vi "7903 Reference Clock Config.vi"(8 "error in":errorcluster, 9 "reference clock index":u8, 10 "ref clk frequency":u64, 11 "fpga interface in":refnum<k20>) -> (0 "error out":errorcluster, 3 "fpga interface out":refnum<k20>)   [LabVIEW 2023, in "PXIe-7903 Aurora Example Host.lvlib"]
uses:
  PXIe-7903 Aurora Example Host.lvlib
  <resource>/objmgr/niflexrioapiClock.rc
  Program Files/NI/LVAddons/flexrioiia/1/instr.lib/FlexRIO/API/Host/v1/NI FlexRIO API v1.lvlib
  <vilib>/ErrorRing/Error Ring.xnode
  <vilib>/Utility/error.llb/Error Cluster From Error Code.vi
  Program Files/NI/LVAddons/flexrioiia/1/instr.lib/FlexRIO/API/Host/v1/NI FlexRIO/API/Get Property Reference - Fpga Small.vi
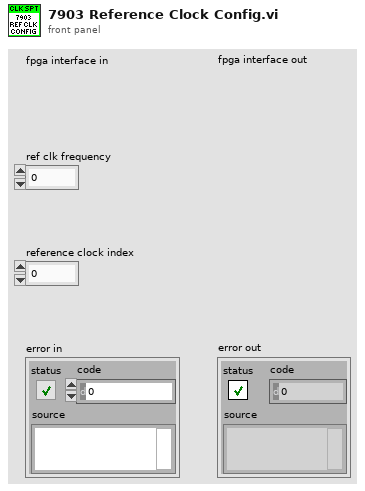
[diagram p1: front panel]
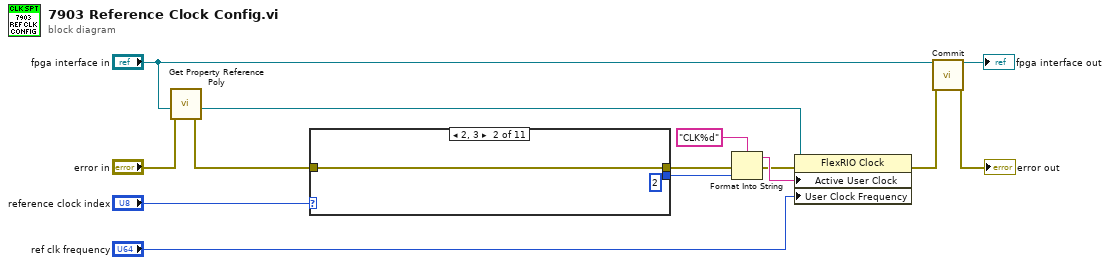
[diagram p0: block diagram]
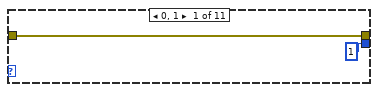
[diagram p2: hidden frame]
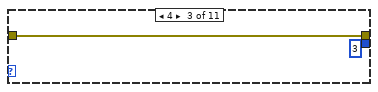
[diagram p3: hidden frame]
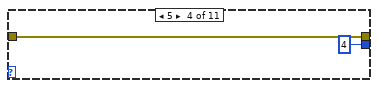
[diagram p4: hidden frame]
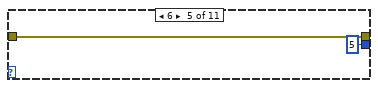
[diagram p5: hidden frame]
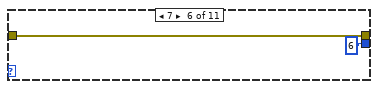
[diagram p6: hidden frame]
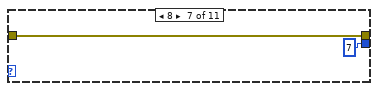
[diagram p7: hidden frame]
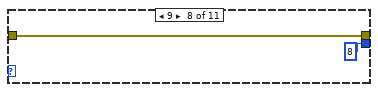
[diagram p8: hidden frame]
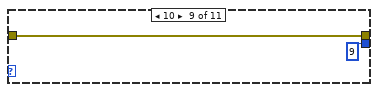
[diagram p9: hidden frame]
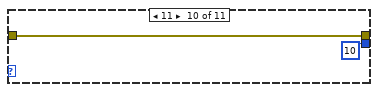
[diagram p10: hidden frame]
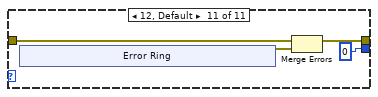
[diagram p11: hidden frame]
diagram:
  n1 = call-poly "Get Property Reference Poly.vi"("error in (no error)"="error in", "fpga interface in"="fpga interface in") -> ("error out"=w4:errorcluster, "property reference"=w14:refnum<k20>)  [unwired: 4 in, 1 out]
  n2 = case shown="2, 3" "reference clock index" {
    tunnel: [u8 1 ("input 1") u8 2 ("input 1") u8 3 ("input 1") u8 4 ("input 1") u8 5 ("input 1") u8 6 ("input 1") u8 7 ("input 1") u8 8 ("input 1") u8 9 ("input 1") u8 10 ("input 1") u8 0 ("input 1")] -> w7
    tunnel: w4 -> [w15 w17 w19 w21 w23 w25 w27 w29 w31 w33 w37]
    tunnel: [w15 w17 w19 w21 w23 w25 w27 w29 w31 w33 w35] -> w3
    frame 0, 1 {
    }
    frame 2, 3 {
    }
    frame 4 {
    }
    frame 5 {
    }
    frame 6 {
    }
    frame 7 {
    }
    frame 8 {
    }
    frame 9 {
    }
    frame 10 {
    }
    frame 11 {
    }
    frame 12, Default {
      n3 = xnode "Error Ring"() -> ("error out"=w36:errorcluster)
      n4 = Merge Errors(w37, w36) -> (w35:errorcluster)
    }
  }
  n5 = Format Into String(format string="CLK%d" ("Active User Clock"), error in=w3, w7) -> (resulting string=w6:string, error out=w5:errorcluster)  [unwired: 1 in]
  n6 = property class="FlexRIO Clock"(reference=w14, error in=w5, "Active User Clock"=w6, "User Clock Frequency"="ref clk frequency") -> (error out=w12:errorcluster)  [unwired: 1 out]
  n7 = call "Commit.vi"("fpga interface in"="fpga interface in", "error in"=w12) -> ("fpga interface out"=→"fpga interface out":refnum<k20>, "error out"=→"error out":errorcluster)  [unwired: 12 in]
